vi "publish.vi"(8 "error in":errorcluster, 9 "timeout":i32, 10 "stream definition":T1, 11 "stream publisher in":refnum<class "data bus stream publisher.lvclass">) -> (0 "error out":errorcluster, 1 "timed out?":bool, 3 "stream publisher out":refnum<class "data bus stream publisher.lvclass">)   [LabVIEW 2013, in "data bus stream publisher.lvclass"]
uses:
  data bus stream publisher.lvclass
  data stream definition.ctl
  data stream message type.ctl
  data bus stream publisher.lvclass/data bus stream publisher.ctl
  subscriber/data bus stream subscriber.lvclass
  subscriber/data bus stream subscriber.lvclass/data bus stream subscriber.ctl
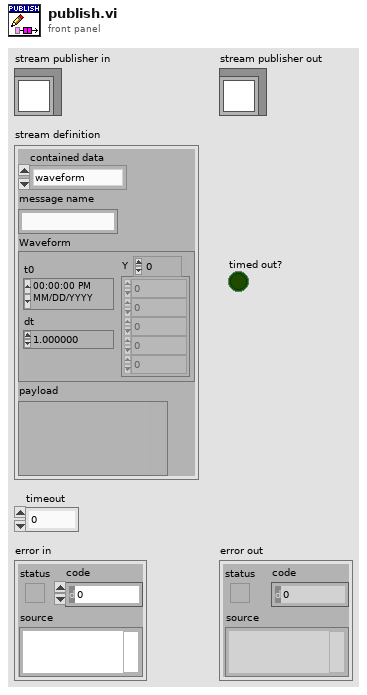
[diagram p1: front panel]
types:
  T1 = typedef "data stream definition.ctl" = cluster{"contained data":T2, "message name":string, "Waveform":waveform(dbl), "payload":variant}
  T2 = typedef "data stream message type.ctl" = enum16{"waveform", "message"}
  T3 = typedef "data bus stream publisher.lvclass/publish mode.ctl" = enum16{"mirror", "round robin"}
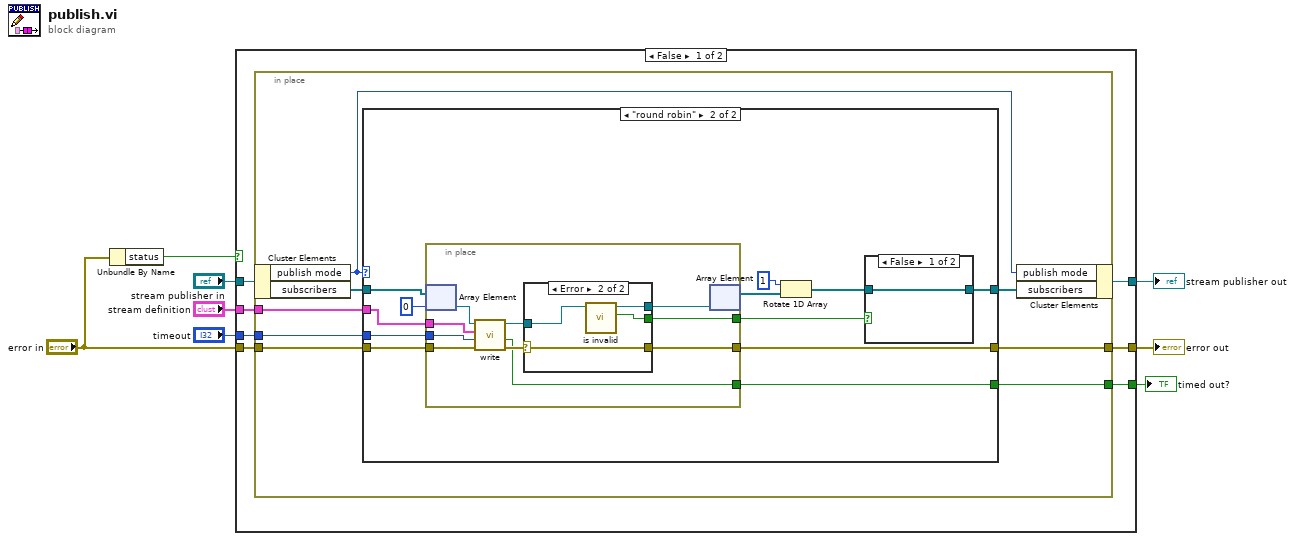
[diagram p0: block diagram]
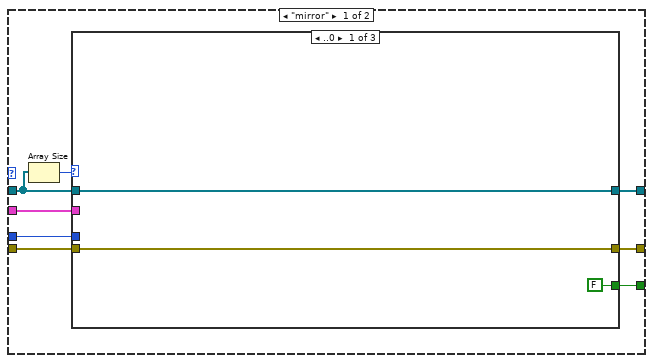
[diagram p2: hidden frame]
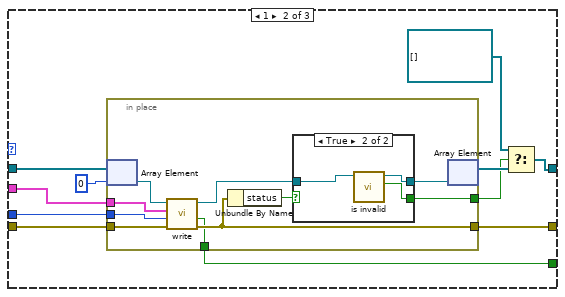
[diagram p3: hidden frame]
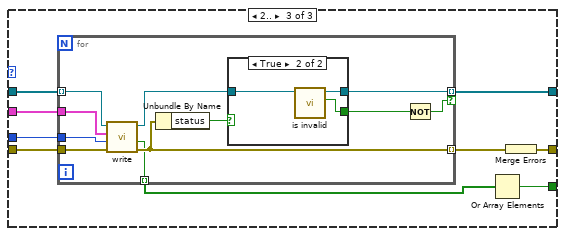
[diagram p5: hidden frame]
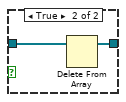
[diagram p7: hidden frame]
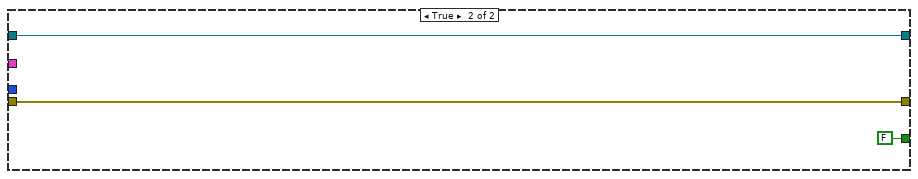
[diagram p9: hidden frame]
diagram:
  n1 = Unbundle By Name("error in") -> ("status"=w2:bool)
  n2 = case shown="False" w2 {
    tunnel: "stream publisher in" -> [w15 w117]
    tunnel: "timeout" -> [w14 _]
    tunnel: "error in" -> [w13 w116]
    tunnel: "stream definition" -> [w12 _]
    tunnel: [w11 w116] -> w5
    tunnel: [w10 w117] -> w4
    tunnel: [w9 FALSE ("timed out?")] -> w1
    frame False {
      n3 = in-place {
        in-place-border: w14 -> [w21]
        in-place-border: w13 -> [w20]
        in-place-border: [w19] -> w11
        in-place-border: w12 -> [w18]
        in-place-border: [w16] -> w9
        n4 = in-place-cluster #1(w15) -> ("publish mode"=w23:T3, "subscribers"=w22:refnum<class "data bus stream subscriber.lvclass">[])
        n5 = case shown="\"round robin\"" w23 {
          tunnel: w22 -> [w29 w95]
          tunnel: w21 -> [w25 w93]
          tunnel: w20 -> [w28 w92]
          tunnel: [w27 w85] -> w19
          tunnel: w18 -> [w26 w91]
          tunnel: [w30 w87] -> w17
          tunnel: [w24 w84] -> w16
          frame "mirror" {
            n6 = Array Size(array=w29) -> (size(s)=w31:i32)
            n7 = case shown="..0" w31 {
              tunnel: [w34 w40 w62] -> w30
              tunnel: w29 -> [w34 w44 w66]
              tunnel: w28 -> [w33 w45 w68]
              tunnel: [w33 w36 w63] -> w27
              tunnel: w26 -> [_ w42 w65]
              tunnel: w25 -> [_ w41 w64]
              tunnel: [FALSE ("timed out?") w35 w60] -> w24
              frame ..0 {
              }
              frame 1 {
                n8 = in-place {
                  in-place-border: w45 -> [w55]
                  in-place-border: [w49] -> w36
                  in-place-border: w42 -> [w53]
                  in-place-border: w41 -> [w52]
                  in-place-border: [w48] -> w37
                  in-place-border: [w46] -> w35
                  n9 = in-place-array #2(w44, 0) -> (w54:refnum<class "data bus stream subscriber.lvclass">)
                  n10 = call "write.vi"("error in"=w55, "timeout in ms (-1)"=w52, "element"=w53, "stream publisher in"=w54) -> ("error out"=w49:errorcluster, "timed out?"=w46:bool, "stream publisher out"=w50:refnum<class "data bus stream subscriber.lvclass">)  [unwired: 5 in]
                  n11 = Unbundle By Name(w49) -> ("status"=w47:bool)
                  n12 = case shown="True" w47 {
                    tunnel: [w56 w58] -> w51
                    tunnel: w50 -> [w56 w59]
                    tunnel: [_ w57] -> w48
                    frame False {
                    }
                    frame True {
                      n13 = call "is invalid.vi"("stream publisher in"=w59) -> ("invalid?"=w57:bool, "stream publisher out"=w58:refnum<class "data bus stream subscriber.lvclass">)  [unwired: 9 in]
                    }
                  }
                  n14 = in-place-array #2(w51) -> (w39:refnum<class "data bus stream subscriber.lvclass">[])  [unwired: 1 out]
                }
                n15 = Select(t=refnum<class "data bus stream subscriber.lvclass">[] [], s=w37, f=w39) -> (s? t:f=w40:refnum<class "data bus stream subscriber.lvclass">[])
              }
              frame 2.. {
                n16 = for {
                  tunnel: w68 -> [w79]
                  tunnel: [w78] -> w67 mode=indexing
                  tunnel: w66 -> [w73] mode=indexing
                  tunnel: w65 -> [w77]
                  tunnel: w64 -> [w76]
                  tunnel: [w72] -> w62 mode=indexing if=w71
                  tunnel: [w69] -> w61 mode=indexing
                  n17 = call "write.vi"("error in"=w79, "timeout in ms (-1)"=w76, "element"=w77, "stream publisher in"=w73) -> ("error out"=w78:errorcluster, "timed out?"=w69:bool, "stream publisher out"=w74:refnum<class "data bus stream subscriber.lvclass">)  [unwired: 5 in]
                  n18 = Unbundle By Name(w78) -> ("status"=w70:bool)
                  n19 = case shown="True" w70 {
                    tunnel: [w80 w82] -> w72
                    tunnel: w74 -> [w80 w83]
                    tunnel: [_ w81] -> w75
                    frame False {
                    }
                    frame True {
                      n20 = call "is invalid.vi"("stream publisher in"=w83) -> ("invalid?"=w81:bool, "stream publisher out"=w82:refnum<class "data bus stream subscriber.lvclass">)  [unwired: 9 in]
                    }
                  }
                  n21 = Not(x=w75) -> (.not. x?=w71:bool)
                }
                n22 = Or Array Elements(Boolean array=w61) -> (logical OR=w60:bool)
                n23 = Merge Errors(w67) -> (w63:errorcluster)
              }
            }
          }
          frame "round robin" {
            n24 = in-place {
              in-place-border: w93 -> [w107]
              in-place-border: w92 -> [w106]
              in-place-border: [w101] -> w85
              in-place-border: w91 -> [w105]
              in-place-border: [w100] -> w88
              in-place-border: [w99] -> w84
              n25 = in-place-array #3(w95, 0) -> (w108:refnum<class "data bus stream subscriber.lvclass">)
              n26 = call "write.vi"("error in"=w106, "timeout in ms (-1)"=w107, "element"=w105, "stream publisher in"=w108) -> ("error out"=w104:errorcluster, "timed out?"=w99:bool, "stream publisher out"=w102:refnum<class "data bus stream subscriber.lvclass">)  [unwired: 5 in]
              n27 = case shown="Error" w104 {
                selector: w104 -> [w109 w112]
                tunnel: [w110 w113] -> w103
                tunnel: w102 -> [w110 w114]
                tunnel: [w109 w112] -> w101
                tunnel: [_ w111] -> w100
                frame No Error {
                }
                frame Error {
                  n28 = call "is invalid.vi"("stream publisher in"=w114) -> ("invalid?"=w111:bool, "stream publisher out"=w113:refnum<class "data bus stream subscriber.lvclass">)  [unwired: 9 in]
                }
              }
              n29 = in-place-array #3(w103) -> (w90:refnum<class "data bus stream subscriber.lvclass">[])  [unwired: 1 out]
            }
            n30 = Rotate 1D Array(1:w90, 2:1 ("n")) -> (0:w86:refnum<class "data bus stream subscriber.lvclass">[])
            n31 = case shown="False" w88 {
              tunnel: [w96 w97] -> w87
              tunnel: w86 -> [w96 w98]
              frame False {
              }
              frame True {
                n32 = Delete From Array(array=w98) -> (array with subset deleted=w97:refnum<class "data bus stream subscriber.lvclass">[])  [unwired: 2 in, 1 out]
              }
            }
          }
        }
        n33 = in-place-cluster #1("publish mode"=w23, "subscribers"=w17) -> (w10:refnum<class "data bus stream publisher.lvclass">)
      }
    }
    frame True {
    }
  }
  "error out" <- w5
  "stream publisher out" <- w4
  "timed out?" <- w1
